vi "Open Log File.vi"(8 "error in (no error)":errorcluster, 11 "Datalogger Object In":refnum<class "Datalogger.lvclass">) -> (0 "error out":errorcluster, 3 "Datalogger Object Out":refnum<class "Datalogger.lvclass">)   [LabVIEW 2018, in "Datalogger.lvlib" / "Datalogger.lvclass"]
uses:
  Datalogger.lvclass
  Datalogger.lvclass/Datalogger.ctl
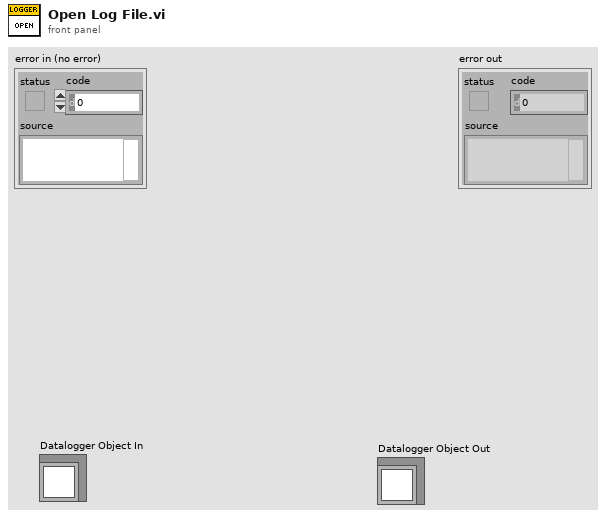
[diagram p1: front panel]
types:
  T1 = enum16{"open", "replace", "create", "open or create", "replace or create", "replace or create with confirmation"}
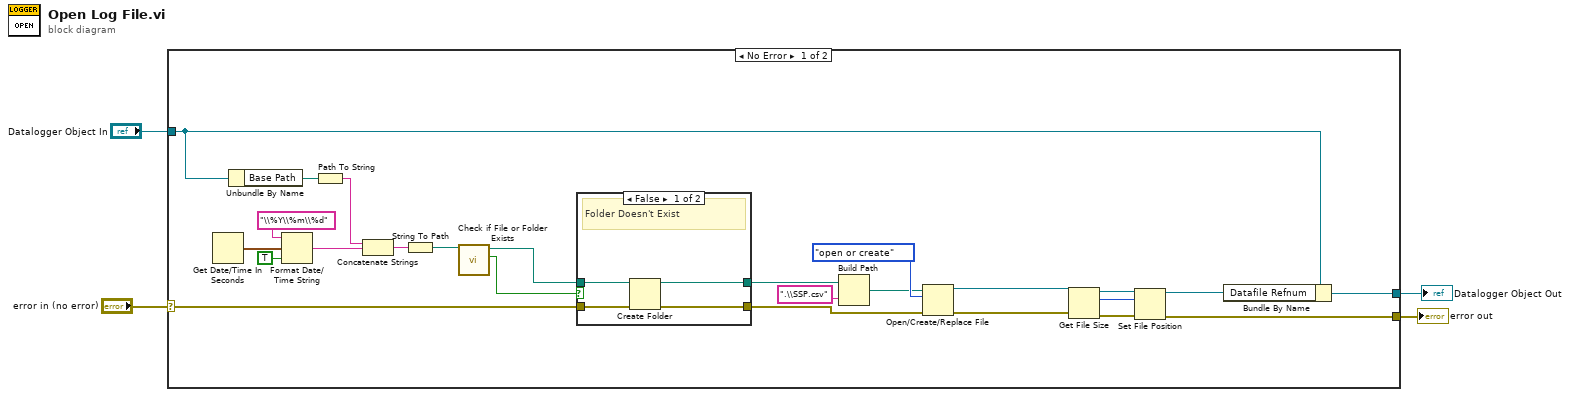
[diagram p0: block diagram]
diagram:
  n1 = case shown="No Error" "error in (no error)" {
    selector: "error in (no error)" -> [w14 w37]
    tunnel: [w8 w37] -> w3
    tunnel: [w20 w36] -> w2
    tunnel: "Datalogger Object In" -> [w21 w36]
    frame No Error {
      n2 = Get Date/Time In Seconds() -> (seconds since 1Jan1904=w25:timestamp)
      n3 = Unbundle By Name(w21) -> ("Base Path"=w29:path)
      n4 = Format Date/Time String(time format string (%c)="\\%Y\\%m\\%d", seconds (now)=w25, UTC format=TRUE) -> (date/time string=w24:string)
      n5 = Path To String(path=w29) -> (string=w28:string)
      n6 = Concatenate Strings(w28, w24) -> (w27:string)
      n7 = String To Path(string=w27) -> (path=w7:path)
      n8 = call <vilib>:"Check if File or Folder Exists.vi"("path"=w7) -> ("file or folder exists?"=w6:bool, "dup path"=w5:path)  [unwired: 8 in, 1 out]
      n9 = case shown="False" w6 {
        tunnel: [w33 w34] -> w18
        tunnel: w14 -> [w32 w35]
        tunnel: [w31 w35] -> w13
        tunnel: w5 -> [w30 w34]
        frame False {
          # "Folder Doesn't Exist"
          n10 = Create Folder(path (use dialog)=w30, error in=w32) -> (created path=w33:path, error out=w31:errorcluster)  [unwired: 1 in, 1 out]
        }
        frame True {
          # "Folder Exists"
        }
      }
      n11 = Build Path(base path=w18, name or relative path=".\\SSP.csv" ("string")) -> (appended path=w17:path)
      n12 = Open/Create/Replace File(file path (use dialog)=w17, error in=w13, operation (0:open)=T1."open or create") -> (refnum out=w16:refnum<file>, error out=w15:errorcluster)  [unwired: 3 in, 1 out]
      n13 = Get File Size(file=w16, error in=w15) -> (refnum out=w10:refnum<file>, size (in bytes)=w11:i64, 0:w12:errorcluster)
      n14 = Set File Position(offset (in bytes) (0)=w11, refnum=w10, error in=w12) -> (refnum out=w9:refnum<file>, error out=w8:errorcluster)  [unwired: 1 in]
      n15 = Bundle By Name(cluster=w21, "Datafile Refnum"=w9) -> (w20:refnum<class "Datalogger.lvclass">)
    }
    frame Error {
    }
  }
  "error out" <- w3
  "Datalogger Object Out" <- w2
